vi "Bai3_2.vi"() -> ()   [LabVIEW 2023]
panel:
  in  "stop":bool
  out "error out":errorcluster
  in  "error in":errorcluster
  in  "DO Lines":bool[](array[boolean])=[FALSE, FALSE, FALSE, FALSE, FALSE, FALSE, FALSE, FALSE]
  in  "Stop":bool=TRUE
  in  "Lines to Write":u16(ring) items=["0 - 7", "8 - 15", "16 - 23"]
  in  "Device Name":tag="Dev8"
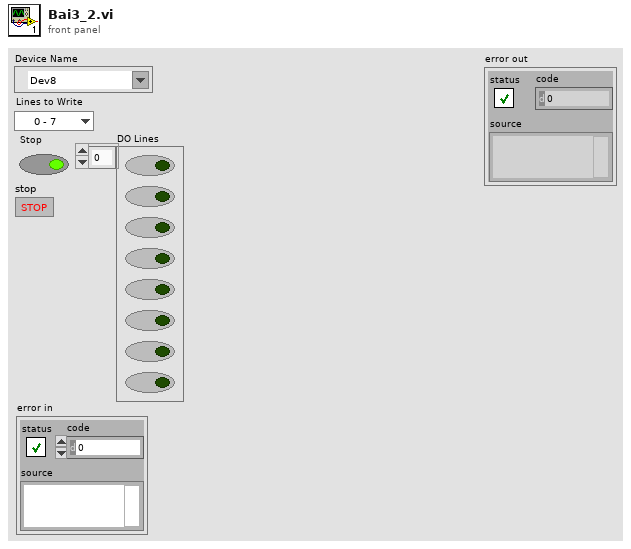
[diagram p1: front panel]
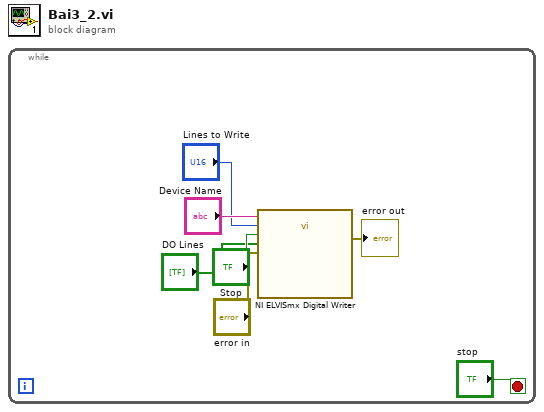
[diagram p0: block diagram]
diagram:
  n1 = while {
    stop <- "stop" stop-if-true
    n2 = call "NI ELVISmx Digital Writer"("Device Name"="Device Name", "Lines to Write"="Lines to Write", "Stop"="Stop", "DO Lines"="DO Lines", "error in"="error in") -> ("error out"=→"error out":errorcluster)  [unwired: 14 in]
  }
